vi "火系攻击.vi"() -> ()   [LabVIEW 2013]
panel:
  in  "簇":T1
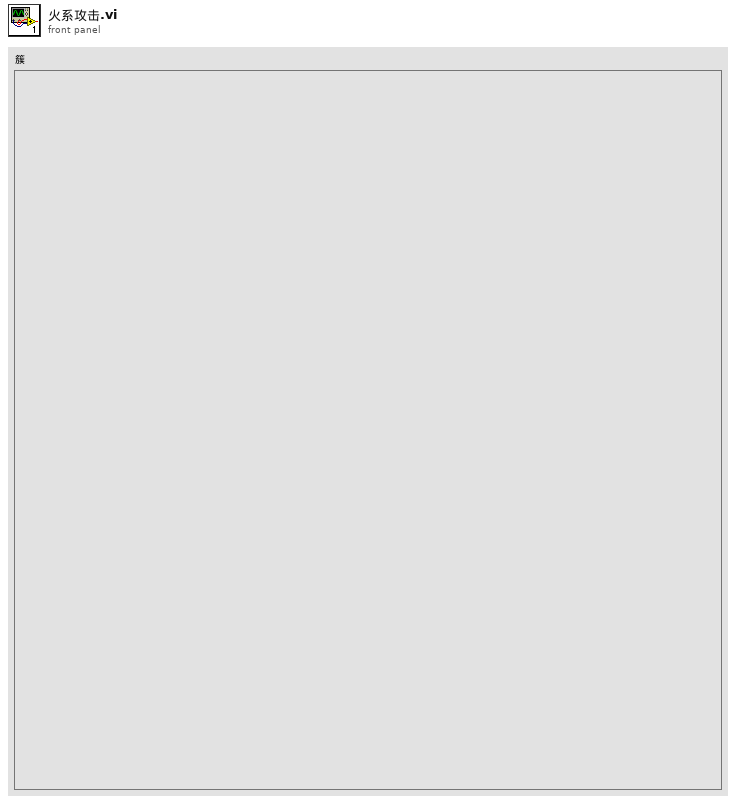
[diagram p1: front panel]
types:
  T1 = cluster{"4":bool, "5":bool, "6":bool, "7":bool, "8":bool, "1":bool, "2":bool, "3":bool, "9":bool, "10":bool, "11":bool, "12":bool, "13":bool, "14":bool, "15":bool, "确定按钮":bool}
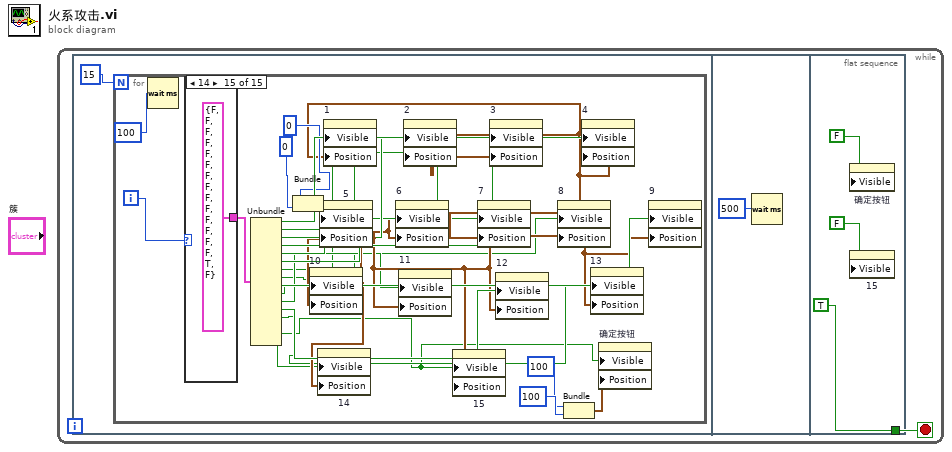
[diagram p0: block diagram]
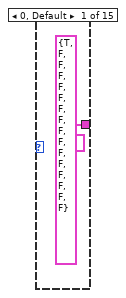
[diagram p2: hidden frame]
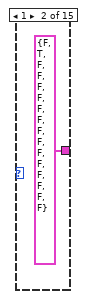
[diagram p3: hidden frame]
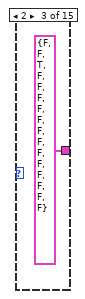
[diagram p4: hidden frame]
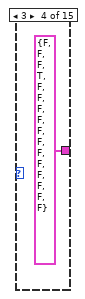
[diagram p5: hidden frame]
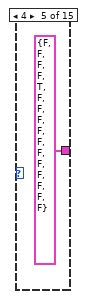
[diagram p6: hidden frame]
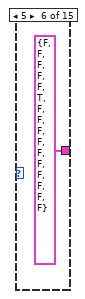
[diagram p7: hidden frame]
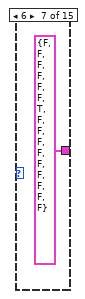
[diagram p8: hidden frame]
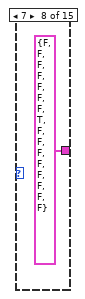
[diagram p9: hidden frame]
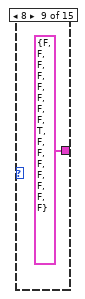
[diagram p10: hidden frame]
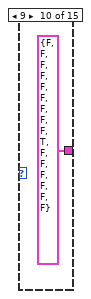
[diagram p11: hidden frame]
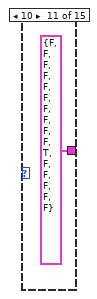
[diagram p12: hidden frame]
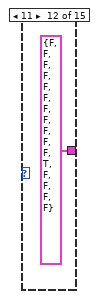
[diagram p13: hidden frame]
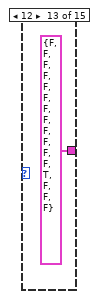
[diagram p14: hidden frame]
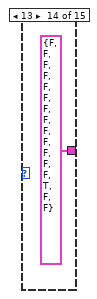
[diagram p15: hidden frame]
diagram:
  n1 = while {
    stop <- w1 stop-if-true
    n2 = flat-sequence {
      tunnel: [TRUE] -> w1
      frame #0 {
        n3 = for {
          N: 15 -> [_]
          i -> [w13]
          n4 = Wait (ms)(milliseconds to wait=100) -> ()  [unwired: 1 out]
          n5 = case shown="14" w13 {
            tunnel: [T1 {"4"=TRUE, "5"=FALSE, "6"=FALSE, "7"=FALSE, "8"=FALSE, "1"=FALSE, "2"=FALSE, "3"=FALSE, "9"=FALSE, "10"=FALSE, "11"=FALSE, "12"=FALSE, "13"=FALSE, "14"=FALSE, "15"=FALSE, "确定按钮"=FALSE} ("簇") T1 {"4"=FALSE, "5"=TRUE, "6"=FALSE, "7"=FALSE, "8"=FALSE, "1"=FALSE, "2"=FALSE, "3"=FALSE, "9"=FALSE, "10"=FALSE, "11"=FALSE, "12"=FALSE, "13"=FALSE, "14"=FALSE, "15"=FALSE, "确定按钮"=FALSE} ("簇") T1 {"4"=FALSE, "5"=FALSE, "6"=TRUE, "7"=FALSE, "8"=FALSE, "1"=FALSE, "2"=FALSE, "3"=FALSE, "9"=FALSE, "10"=FALSE, "11"=FALSE, "12"=FALSE, "13"=FALSE, "14"=FALSE, "15"=FALSE, "确定按钮"=FALSE} ("簇") T1 {"4"=FALSE, "5"=FALSE, "6"=FALSE, "7"=TRUE, "8"=FALSE, "1"=FALSE, "2"=FALSE, "3"=FALSE, "9"=FALSE, "10"=FALSE, "11"=FALSE, "12"=FALSE, "13"=FALSE, "14"=FALSE, "15"=FALSE, "确定按钮"=FALSE} ("簇") T1 {"4"=FALSE, "5"=FALSE, "6"=FALSE, "7"=FALSE, "8"=TRUE, "1"=FALSE, "2"=FALSE, "3"=FALSE, "9"=FALSE, "10"=FALSE, "11"=FALSE, "12"=FALSE, "13"=FALSE, "14"=FALSE, "15"=FALSE, "确定按钮"=FALSE} ("簇") T1 {"4"=FALSE, "5"=FALSE, "6"=FALSE, "7"=FALSE, "8"=FALSE, "1"=TRUE, "2"=FALSE, "3"=FALSE, "9"=FALSE, "10"=FALSE, "11"=FALSE, "12"=FALSE, "13"=FALSE, "14"=FALSE, "15"=FALSE, "确定按钮"=FALSE} ("簇") T1 {"4"=FALSE, "5"=FALSE, "6"=FALSE, "7"=FALSE, "8"=FALSE, "1"=FALSE, "2"=TRUE, "3"=FALSE, "9"=FALSE, "10"=FALSE, "11"=FALSE, "12"=FALSE, "13"=FALSE, "14"=FALSE, "15"=FALSE, "确定按钮"=FALSE} ("簇") T1 {"4"=FALSE, "5"=FALSE, "6"=FALSE, "7"=FALSE, "8"=FALSE, "1"=FALSE, "2"=FALSE, "3"=TRUE, "9"=FALSE, "10"=FALSE, "11"=FALSE, "12"=FALSE, "13"=FALSE, "14"=FALSE, "15"=FALSE, "确定按钮"=FALSE} ("簇") T1 {"4"=FALSE, "5"=FALSE, "6"=FALSE, "7"=FALSE, "8"=FALSE, "1"=FALSE, "2"=FALSE, "3"=FALSE, "9"=TRUE, "10"=FALSE, "11"=FALSE, "12"=FALSE, "13"=FALSE, "14"=FALSE, "15"=FALSE, "确定按钮"=FALSE} ("簇") T1 {"4"=FALSE, "5"=FALSE, "6"=FALSE, "7"=FALSE, "8"=FALSE, "1"=FALSE, "2"=FALSE, "3"=FALSE, "9"=FALSE, "10"=TRUE, "11"=FALSE, "12"=FALSE, "13"=FALSE, "14"=FALSE, "15"=FALSE, "确定按钮"=FALSE} ("簇") T1 {"4"=FALSE, "5"=FALSE, "6"=FALSE, "7"=FALSE, "8"=FALSE, "1"=FALSE, "2"=FALSE, "3"=FALSE, "9"=FALSE, "10"=FALSE, "11"=TRUE, "12"=FALSE, "13"=FALSE, "14"=FALSE, "15"=FALSE, "确定按钮"=FALSE} ("簇") T1 {"4"=FALSE, "5"=FALSE, "6"=FALSE, "7"=FALSE, "8"=FALSE, "1"=FALSE, "2"=FALSE, "3"=FALSE, "9"=FALSE, "10"=FALSE, "11"=FALSE, "12"=TRUE, "13"=FALSE, "14"=FALSE, "15"=FALSE, "确定按钮"=FALSE} ("簇") T1 {"4"=FALSE, "5"=FALSE, "6"=FALSE, "7"=FALSE, "8"=FALSE, "1"=FALSE, "2"=FALSE, "3"=FALSE, "9"=FALSE, "10"=FALSE, "11"=FALSE, "12"=FALSE, "13"=TRUE, "14"=FALSE, "15"=FALSE, "确定按钮"=FALSE} ("簇") T1 {"4"=FALSE, "5"=FALSE, "6"=FALSE, "7"=FALSE, "8"=FALSE, "1"=FALSE, "2"=FALSE, "3"=FALSE, "9"=FALSE, "10"=FALSE, "11"=FALSE, "12"=FALSE, "13"=FALSE, "14"=TRUE, "15"=FALSE, "确定按钮"=FALSE} ("簇") T1 {"4"=FALSE, "5"=FALSE, "6"=FALSE, "7"=FALSE, "8"=FALSE, "1"=FALSE, "2"=FALSE, "3"=FALSE, "9"=FALSE, "10"=FALSE, "11"=FALSE, "12"=FALSE, "13"=FALSE, "14"=FALSE, "15"=TRUE, "确定按钮"=FALSE} ("簇")] -> w12
            frame 0, Default {
            }
            frame 1 {
            }
            frame 2 {
            }
            frame 3 {
            }
            frame 4 {
            }
            frame 5 {
            }
            frame 6 {
            }
            frame 7 {
            }
            frame 8 {
            }
            frame 9 {
            }
            frame 10 {
            }
            frame 11 {
            }
            frame 12 {
            }
            frame 13 {
            }
            frame 14 {
            }
          }
          n6 = Unbundle(w12) -> ("4"=w25:bool, "5"=w24:bool, "6"=w23:bool, "7"=w22:bool, "8"=w21:bool, "1"=w20:bool, "2"=w8:bool, "3"=w7:bool, "9"=w17:bool, "10"=w16:bool, "11"=w11:bool, "12"=w15:bool, "13"=w5:bool, "14"=w6:bool, "15"=w3:bool)  [unwired: 1 out]
          n7 = Bundle(0, 0) -> (w14:cluster{i32, i32})  [unwired: 1 in]
          n8 = property on="10" class="Bool"("Visible"=w16, "Position"=w14) -> ()  [unwired: 2 in, 2 out]
          n9 = property on="14" class="Bool"("Visible"=w6, "Position"=w14) -> ()  [unwired: 2 in, 2 out]
          n10 = property on="5" class="Bool"("Visible"=w21, "Position"=w14) -> ()  [unwired: 2 in, 2 out]
          n11 = property on="1" class="Bool"("Visible"=w25, "Position"=w14) -> ()  [unwired: 2 in, 2 out]
          n12 = property on="6" class="Bool"("Visible"=w20, "Position"=w14) -> ()  [unwired: 2 in, 2 out]
          n13 = property on="11" class="Bool"("Visible"=w11, "Position"=w14) -> ()  [unwired: 2 in, 2 out]
          n14 = property on="2" class="Bool"("Visible"=w24, "Position"=w14) -> ()  [unwired: 2 in, 2 out]
          n15 = property on="15" class="Bool"("Visible"=w3, "Position"=w14) -> ()  [unwired: 2 in, 2 out]
          n16 = property on="7" class="Bool"("Visible"=w8, "Position"=w14) -> ()  [unwired: 2 in, 2 out]
          n17 = property on="3" class="Bool"("Visible"=w23, "Position"=w14) -> ()  [unwired: 2 in, 2 out]
          n18 = property on="12" class="Bool"("Visible"=w15, "Position"=w14) -> ()  [unwired: 2 in, 2 out]
          n19 = property on="8" class="Bool"("Visible"=w7, "Position"=w14) -> ()  [unwired: 2 in, 2 out]
          n20 = Bundle(100, 100) -> (w4:cluster{i32, i32})  [unwired: 1 in]
          n21 = property on="4" class="Bool"("Visible"=w22, "Position"=w14) -> ()  [unwired: 2 in, 2 out]
          n22 = property on="13" class="Bool"("Visible"=w5, "Position"=w14) -> ()  [unwired: 2 in, 2 out]
          n23 = property on="确定按钮" class="Bool"("Visible"=w3, "Position"=w4) -> ()  [unwired: 2 in, 2 out]
          n24 = property on="9" class="Bool"("Visible"=w17, "Position"=w14) -> ()  [unwired: 2 in, 2 out]
        }
      }
      frame #1 {
        n25 = Wait (ms)(milliseconds to wait=500) -> ()  [unwired: 1 out]
      }
      frame #2 {
        n26 = property on="确定按钮" class="Bool"("Visible"=FALSE) -> ()  [unwired: 2 in, 2 out]
        n27 = property on="15" class="Bool"("Visible"=FALSE) -> ()  [unwired: 2 in, 2 out]
      }
    }
  }
